vi "threshold_init.vi"(0 "reg_max":refnum<k21>, 1 "max":fxp<+,16,8>, 2 "min":fxp<+,16,8>, 3 "reg_min":refnum<k21>, 4 "Enable":bool) -> (5 "Register Out":refnum<k21>, 7 "Register Out 2":refnum<k21>)   [LabVIEW 2018]
uses:
  <vilib>/rvi/DataTransferAndStorage/Container/XNode/niFpgaContainer.xnode
  <vilib>/rvi/DataTransferAndStorage/Register/Emulation/niFpgaRegisterEmulationRefIn.vi
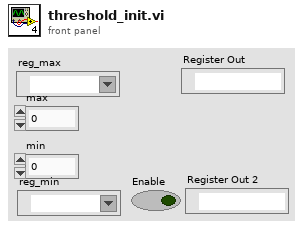
[diagram p1: front panel]
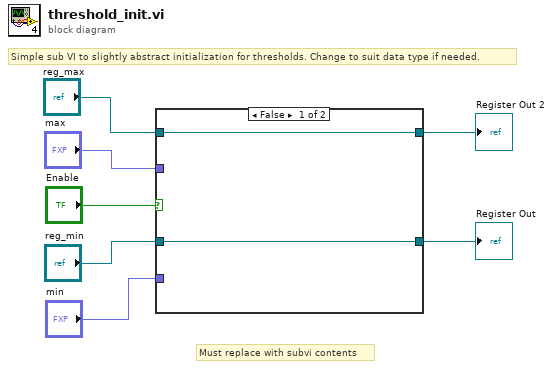
[diagram p0: block diagram]
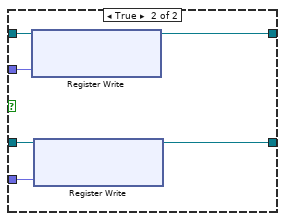
[diagram p2: hidden frame]
diagram:
  # "Must replace with subvi contents"
  # "Simple sub VI to slightly abstract initialization for thresholds. Change to suit data type if needed."
  n1 = case shown="False" "Enable" {
    tunnel: "reg_max" -> [w9 w15]
    tunnel: "reg_min" -> [w8 w14]
    tunnel: "max" -> [_ w13]
    tunnel: "min" -> [_ w12]
    tunnel: [w9 w11] -> w3
    tunnel: [w8 w10] -> w2
    frame False {
    }
    frame True {
      n2 = xnode "Register Write"("Data"=w13, "Register In"=w15) -> ("Register Out"=w11:refnum<k21>)
      n3 = xnode "Register Write"("Data"=w12, "Register In"=w14) -> ("Register Out"=w10:refnum<k21>)
    }
  }
  "Register Out" <- w2
  "Register Out 2" <- w3
